vi "Do.vi"(8 "error in":errorcluster, 10 "Actor in":refnum<class "Actor.lvclass">, 11 "Enable Channel 1 Laser":refnum<class "Update PAS Laser 1 Enable State MSG.lvclass">) -> (0 "error out":errorcluster, 2 "Actor out":refnum<class "Actor.lvclass">)   [LabVIEW 2017, in "Controller.lvlib" / "Update PAS Laser 1 Enable State MSG.lvclass"]
doc: "(<B>Filename</B>: Actor Framework.lvlib:Message.lvclass:Do.vi)\n\nDefines what a message does when it is received by an actor. Generally, a message instructs an actor to invoke one of its methods. By default, this method does nothing. A child class must override it to define behavior. Create a child class by using the Actor Framework Message Maker dialog box."
uses:
  Update PAS Laser 1 Enable State MSG.lvclass
  W:/sw_repo/For Builds/Nicholas/Controller/Messages/Generic Boolean MSG/Generic Boolean Message.lvclass
  <vilib>/ActorFramework/Actor/Actor.lvclass
  Global FPGA DO.ctl
  Generic Boolean MSG/Generic Boolean Message.lvclass/Generic Boolean Message.ctl
  Generic Boolean MSG/Read Bool.vi
  <vilib>/Utility/error.llb/Error Cluster From Error Code.vi
  <vilib>/rvi/errors/niLvFpgaAdjustHostInterfaceError.vi
  Global DO.vi
  <vilib>/rvi/interface/nirviReadWriteControl/nirviReadWriteControl.xnode
  FPGA Ref.ctl
  FPGA Bitfiles/server.lvbitx
  gController.lvclass
  NiFpgaLv.dll
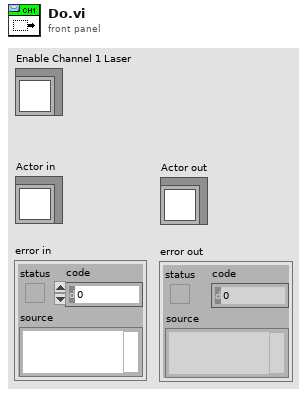
[diagram p1: front panel]
types:
  T1 = typedef "Global FPGA DO.ctl" = enum16{"pas_laser_relay_1", "pas_heater_1", "pas_heater_2", "pas_laser_relay_2", "pas_spk_enable_1", "pas_spk_enable_2", "hanbay_pos", "fan_enable", "crd_laser_enable", "crd_heater_enable", "vacuum_pump", "ac_spare", "uv_enable", "solenoid_1", "solenoid_2", "spare_dc_relay_1", "usb_hub_relay", "spare_dc_relay_2", "fp_aux_1", "fp_aux_2"}
  T2 = typedef "FPGA Ref.ctl" = refnum<k20>
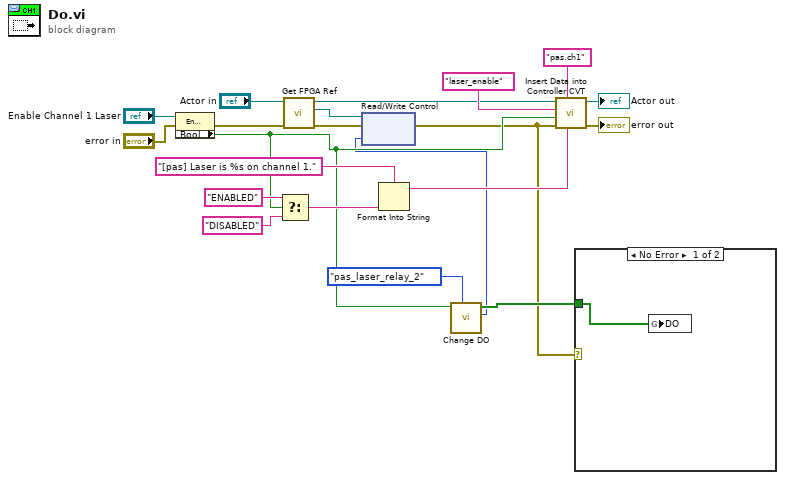
[diagram p0: block diagram]
diagram:
  n1 = property class="Enable PAS Laser 1"(reference="Enable Channel 1 Laser", error in="error in") -> (error out=w7:errorcluster, "Bool"=w3:bool)  [unwired: 1 out]
  n2 = Select(t="ENABLED", s=w3, f="DISABLED") -> (s? t:f=w14:string)
  n3 = call "Get FPGA Ref.vi"("error in (no error)"=w7, "Actor In"="Actor in") -> ("error out"=w6:errorcluster, "FPGA Ref"=w9:T2, "Actor Out"=w10:refnum<class "Actor.lvclass">)  [unwired: 7 in]
  n4 = Format Into String(format string="[pas] Laser is %s on channel 1.", w14) -> (resulting string=w12:string)  [unwired: 2 in, 1 out]
  n5 = call "Change DO.vi"("DO"=Global_FPGA_DO."pas_laser_relay_2", "val_in"=w3) -> ("DO Long Out"=w1:u32, "DO Out"=w4:bool[])  [unwired: 8 in]
  n6 = xnode "Read/Write Control"("FPGA VI Reference In"=w9, "error in"=w6, "DO"=w1) -> ("error out"=w2:errorcluster)  [unwired: 1 out]
  n7 = call "Insert Data into Controller CVT.vi"("Update MSG"=w12, "Group"="pas.ch1", "error in"=w2, "Data"=w3, "tag"="laser_enable", "Actor in"=w10) -> ("error out"=→"error out":errorcluster, "Actor Out"=→"Actor out":refnum<class "Actor.lvclass">)  [unwired: 4 in]
  n8 = case shown="No Error" w2 {
    tunnel: w4 -> [w22 _]
    frame No Error {
      n9 = global write "Global DO.vi" "DO"(w22) -> ()
    }
    frame Error {
    }
  }
